vi "TX.vi"() -> ()   [LabVIEW 2020]
uses:
  AppData/Local/Programs/Python/Python35-32/Control 1.ctl
  <vilib>/Analysis/2dsp.llb/1D Convolution (DBL).vi
  <vilib>/Analysis/baseanly.llb/Quick Scale 1D.vi
  <vilib>/addons/Modulation/Analog/support/mod_Set Error Source.vi
  <vilib>/Enthought/Python Integration Toolkit/api/Unpack Int Array.vi
  <vilib>/addons/Modulation/Digital/Support/Common/Validators/mod_Generate Filter Coefficients Validate.vi
  <vilib>/addons/Modulation/Digital/General/subVIs/mod_Generate Filter Coefficients.vi
  <vilib>/Analysis/2dsp.llb/Upsample (DBL).vi
  <vilib>/measure/maspectr.llb/FFT Power Spectrum and PSD for 1 Chan (CDB).vi
  <instrlib>/niUSRP/niUSRP Write Tx Data (CDB Cluster).vi
  <vilib>/Analysis/NI_AALPro.lvlib
  <vilib>/measure/NI_MAPro.lvlib
  <vilib>/addons/Modulation/niDMT.lvlib
  <vilib>/Analysis/NI_AALBase.lvlib
  <vilib>/Enthought/Python Integration Toolkit/Python Integration Toolkit.lvlib
panel:
  in  "file path (use dialog)":path=path "C:/Users/ira_1/AppData/Local/Programs/Python/Python35-32/samples.txt"
  in  "Write sample file":bool
  in  "Timeout":dbl=10.0
  in  "Stop":bool
  in  "stop":bool
  in  "active antenna":string="TX1"
  out "Waveform Graph 2":cluster{"f0":dbl, "df":dbl, "magnitude":dbl[]}(graph)
  out "Waveform Graph":waveform(dbl)(graph)
  in  "averaging parameters":T1={"averaging mode"=enum."No averaging", "weighting mode"=enum."Exponential", "number of averages"=10} {"number of averages" min=1}
  in  "Delay":dbl
  out "error out":errorcluster
  out "Value":i32[](array[numeric])
  out "Кол-во символов":dbl
  in  "speed symbols(sym/sec)":dbl=1023000.0
  in  "NKA id":dbl=1.0
  in  "Doppler":dbl
  out "coerced gain(dB":dbl
  out "coerced carrier frequency":dbl
  out "coerced IQ rate":dbl
  in  "USRP name":T2="B200"
  in  "IQ rate(дискретизацтя)":dbl=4092000.0
  in  "Gain(dB)":dbl=-10.0
  in  "Freq":dbl=1575450000.0
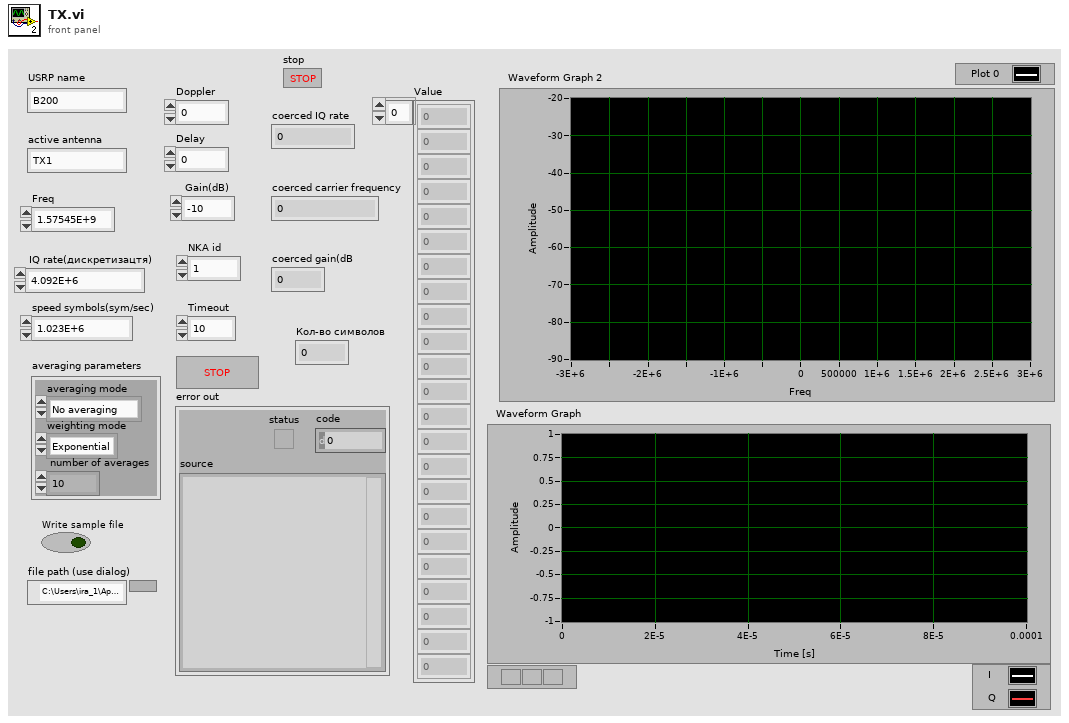
[diagram p1: front panel]
types:
  T1 = cluster{"averaging mode":enum16{"No averaging", "Vector averaging", "RMS averaging", "Peak hold"}, "weighting mode":enum16{"Linear", "Exponential"}, "number of averages":u32}
  T2 = typedef "Control 1.ctl" = string
  T3 = enum16{"none", "Raised Cosine", "Root Raised Cos", "Gaussian"}
  T4 = enum16{"FSK", "PSK", "QAM", "MSK", "PAM", "ASK", "CPM"}
  T5 = enum16{"open", "replace", "create", "open or create", "replace or create", "replace or create with confirmation"}
  T6 = typedef "Python Integration Toolkit.lvlib/Session ID.ctl" = u64
  T7 = typedef "Python Integration Toolkit.lvlib/Python Objects.ctl" = variant
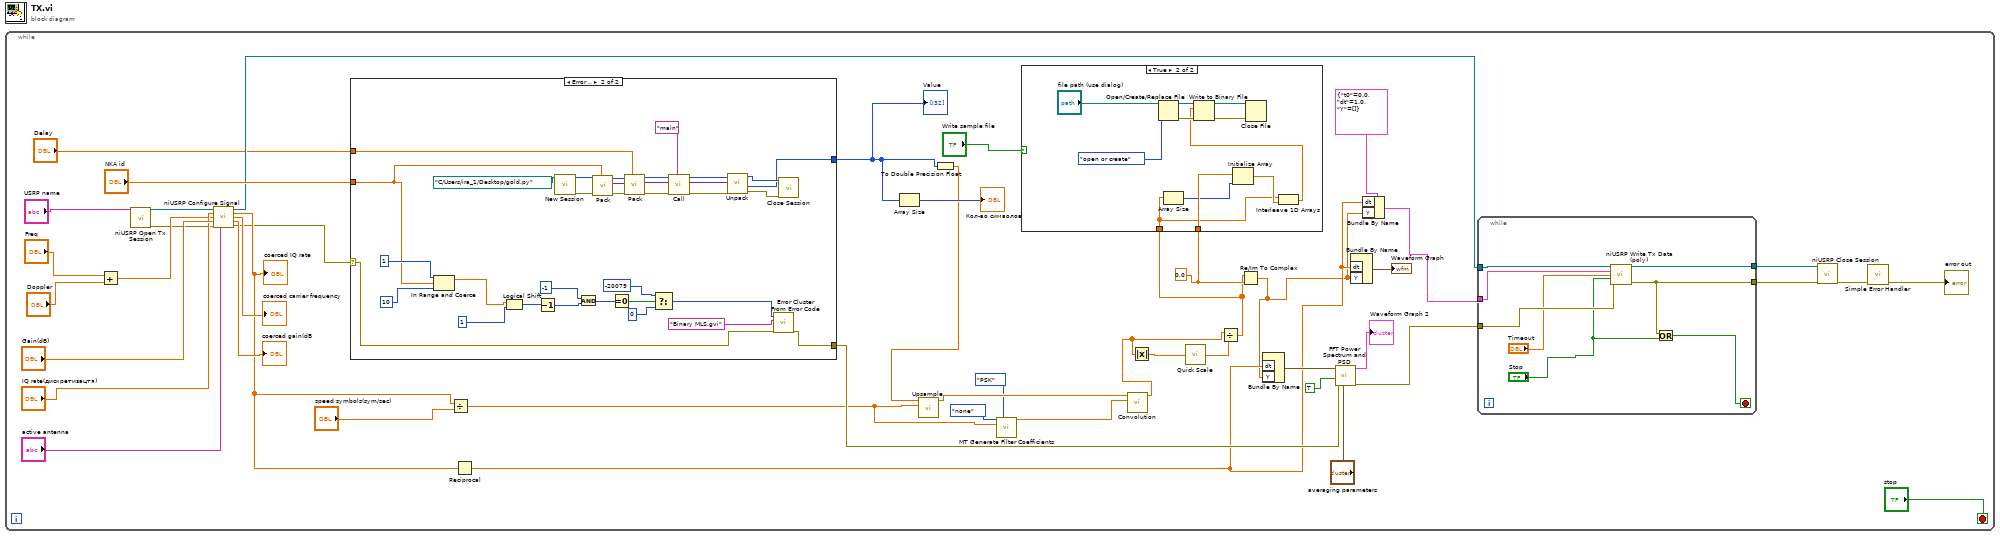
[diagram p0: block diagram]
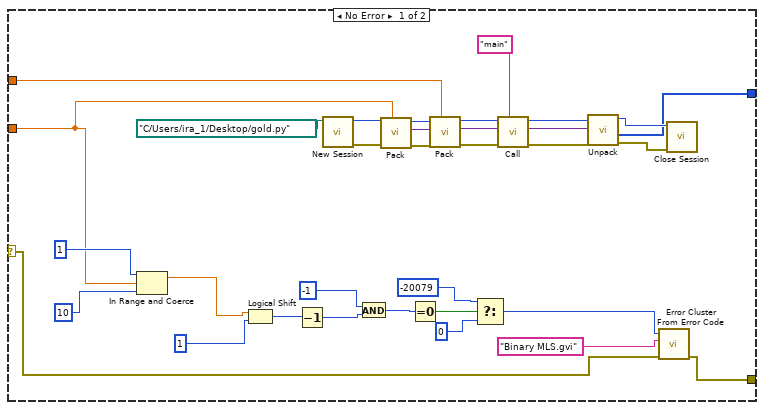
[diagram p3: hidden frame]
diagram:
  n1 = while {
    stop <- "stop" stop-if-true
    w3 = 0.0
    n2 = Add(x="Freq", y="Doppler") -> (x+y=w39:dbl)
    n3 = call <instrlib>:"niUSRP Open Tx Session.vi"("device names"="USRP name") -> ("session handle out"=w46:refnum<k15>, "error out"=w13:errorcluster)  [unwired: 13 in]
    n4 = call <instrlib>:"niUSRP Configure Signal.vi"("session handle"=w46, "IQ rate"="IQ rate(дискретизацтя)", "carrier frequency"=w39, "gain"="Gain(dB)", "error in (no error)"=w13, "active antenna"="active antenna") -> ("session handle out"=w25:refnum<k15>, "coerced IQ rate"=w36:dbl, "coerced carrier frequency"=→"coerced carrier frequency":dbl, "coerced gain"=→"coerced gain(dB":dbl, "error out"=w8:errorcluster)  [unwired: 5 in]
    "coerced IQ rate" <- w36
    n5 = case shown="Error .." w8 {
      selector: w8 -> [w67 w100]
      tunnel: "NKA id" -> [w69 w102]
      tunnel: [w86 w119] -> w32
      tunnel: [w75 w108] -> w34
      tunnel: "Delay" -> [w68 w101]
      frame No Error {
        n6 = In Range and Coerce(upper limit=1, x=w69, lower limit=10) -> (coerced(x)=w96:dbl)  [unwired: 1 out]
        n7 = Logical Shift(y=w96, x=1) -> (x << y=w95:i32)
        n8 = Decrement(x=w95) -> (x-1=w94:i32)
        n9 = call <vilib>:"New Session.vi"("Path to Python Module (.py File)"=path "C:/Users/ira_1/Desktop/gold.py") -> ("error out"=w73:errorcluster, "Session ID out"=w74:T6)  [unwired: 9 in]
        n10 = And(x=-1, y=w94) -> (x .and. y?=w92:i32)
        n11 = call <vilib>:"Pack.vi"("Argument"=w69, "error in (no error)"=w73, "Session ID"=w74) -> ("error out"=w72:errorcluster, "Python Object References Out"=w70:T7, "Session ID out"=w71:T6)  [unwired: 6 in]
        n12 = Equal To 0?(x=w92) -> (x = 0?=w91:bool)
        n13 = call <vilib>:"Pack.vi"("Argument"=w68, "error in (no error)"=w72, "Python Object References In"=w70, "Session ID"=w71) -> ("error out"=w79:errorcluster, "Python Object References Out"=w76:T7, "Session ID out"=w85:T6)  [unwired: 5 in]
        n14 = Select(t=-20079, s=w91, f=0) -> (s? t:f=w87:i32)
        n15 = call <vilib>:"Call.vi"("Function or Method Name"="main", "error in (no error)"=w79, "Python Object References In"=w76, "Session ID"=w85) -> ("error out"=w80:errorcluster, "Python Object References Out"=w81:T7, "Session ID out"=w84:T6)  [unwired: 5 in]
        n16 = call-poly <vilib>:"Unpack.vi"("error in (no error)"=w80, "Python Object References In"=w81, "Session ID"=w84) -> ("error out"=w82:errorcluster, "Value"=w75:i32[], "Session ID out"=w83:T6)  [unwired: 5 in, 1 out]
        n17 = call <vilib>:"Error Cluster From Error Code.vi"("error in (no error)"=w67, "error message (\"\")"="Binary MLS.gvi", "error code (0)"=w87) -> ("error out"=w86:errorcluster)  [unwired: 6 in]
        n18 = call <vilib>:"Close Session.vi"("error in (no error)"=w82, "Session ID"=w83) -> ()  [unwired: 9 in, 1 out]
      }
      frame Error {
        n19 = In Range and Coerce(upper limit=1, x=w102, lower limit=10) -> (coerced(x)=w129:dbl)  [unwired: 1 out]
        n20 = Logical Shift(y=w129, x=1) -> (x << y=w128:i32)
        n21 = Decrement(x=w128) -> (x-1=w127:i32)
        n22 = call <vilib>:"New Session.vi"("Path to Python Module (.py File)"=path "C:/Users/ira_1/Desktop/gold.py") -> ("error out"=w106:errorcluster, "Session ID out"=w107:T6)  [unwired: 9 in]
        n23 = And(x=-1, y=w127) -> (x .and. y?=w125:i32)
        n24 = call <vilib>:"Pack.vi"("Argument"=w102, "error in (no error)"=w106, "Session ID"=w107) -> ("error out"=w105:errorcluster, "Python Object References Out"=w103:T7, "Session ID out"=w104:T6)  [unwired: 6 in]
        n25 = Equal To 0?(x=w125) -> (x = 0?=w124:bool)
        n26 = call <vilib>:"Pack.vi"("Argument"=w101, "error in (no error)"=w105, "Python Object References In"=w103, "Session ID"=w104) -> ("error out"=w112:errorcluster, "Python Object References Out"=w109:T7, "Session ID out"=w118:T6)  [unwired: 5 in]
        n27 = Select(t=-20079, s=w124, f=0) -> (s? t:f=w120:i32)
        n28 = call <vilib>:"Call.vi"("Function or Method Name"="main", "error in (no error)"=w112, "Python Object References In"=w109, "Session ID"=w118) -> ("error out"=w113:errorcluster, "Python Object References Out"=w114:T7, "Session ID out"=w117:T6)  [unwired: 5 in]
        n29 = call-poly <vilib>:"Unpack.vi"("error in (no error)"=w113, "Python Object References In"=w114, "Session ID"=w117) -> ("error out"=w115:errorcluster, "Value"=w108:i32[], "Session ID out"=w116:T6)  [unwired: 5 in, 1 out]
        n30 = call <vilib>:"Error Cluster From Error Code.vi"("error in (no error)"=w100, "error message (\"\")"="Binary MLS.gvi", "error code (0)"=w120) -> ("error out"=w119:errorcluster)  [unwired: 6 in]
        n31 = call <vilib>:"Close Session.vi"("error in (no error)"=w115, "Session ID"=w116) -> ()  [unwired: 9 in, 1 out]
      }
    }
    "Value" <- w34
    n32 = Divide(x=w36, y="speed symbols(sym/sec)") -> (x/y=w23:dbl)
    n33 = Reciprocal(x=w36) -> (1/x=w12:dbl)
    n34 = Array Size(array=w34) -> (size(s)=→"Кол-во символов":i32)
    n35 = To Double Precision Float(number=w34) -> (double precision float=w33:dbl[])
    n36 = call-poly <vilib>:"Upsample.vi"("upsampling factor"=w23, "X"=w33) -> ("Upsampled Array"=w21:dbl[])  [unwired: 8 in, 1 out]
    n37 = call <vilib>:"MT Generate Filter Coefficients.vi"("pulse shaping filter (none)"=T3."none", "modulation type"=T4."PSK", "pulse shaping samples per symbol (16)"=w23) -> ("pulse shaping filter coefficients"=w22:dbl[])  [unwired: 10 in, 2 out]
    n38 = call-poly <vilib>:"Convolution.vi"("Y"=w22, "X"=w21) -> ("X * Y"=w18:dbl[])  [unwired: 8 in, 1 out]
    n39 = Absolute Value(x=w18) -> (abs(x)=w15:dbl[])
    n40 = call-poly <vilib>:"Quick Scale.vi"("X"=w15) -> ("max|X|"=w14:dbl)  [unwired: 2 out]
    n41 = Divide(x=w18, y=w14) -> (x/y=w2:dbl[])
    n42 = case shown="True" "Write sample file" {
      tunnel: w3 -> [_ w58]
      tunnel: w2 -> [_ w50]
      frame False {
      }
      frame True {
        n43 = Open/Create/Replace File(file path (use dialog)="file path (use dialog)", operation (0:open)=T5."open or create") -> (refnum out=w55:refnum<file>, error out=w54:errorcluster)  [unwired: 4 in, 1 out]
        n44 = Array Size(array=w50) -> (size(s)=w57:i32)
        n45 = Initialize Array(w58, w57) -> (w56:dbl[])
        n46 = Interleave 1D Arrays(w50, w56) -> (w53:dbl[])
        n47 = Write to Binary File(file (use dialog)=w55, data=w53, error in=w54) -> (refnum out=w51:refnum<file>, error out=w52:errorcluster)  [unwired: 3 in, 1 out]
        n48 = Close File(refnum=w51, error in=w52) -> ()  [unwired: 2 out]
      }
    }
    n49 = Re/Im To Complex(1:w3, 2:w2) -> (0:w4:cdb[])
    n50 = Bundle By Name("dt"=w12, "Y"=w4) -> (w17:waveform(cdb))  [unwired: 1 in]
    n51 = call-poly <vilib>:"FFT Power Spectrum and PSD.vi"("averaging parameters"="averaging parameters", "error in (no error)"=w32, "dB On (F)"=TRUE, "time signal"=w17) -> ("error out"=w30:errorcluster, "Power Spectrum / PSD"=→"Waveform Graph 2":cluster{"f0":dbl, "df":dbl, "magnitude":dbl[]})  [unwired: 4 in, 2 out]
    n52 = Bundle By Name("dt"=w12, "Y"=w4) -> (→"Waveform Graph":waveform(cdb))  [unwired: 1 in]
    n53 = Bundle By Name(cluster=cluster{"t0":dbl, "dt":dbl, "Y":cdb[]} {"t0"=0.0, "dt"=1.0, "Y"=[]} ("data"), "dt"=w12, "Y"=w4) -> (w11:cluster{"t0":dbl, "dt":dbl, "Y":cdb[]})
    n54 = while {
      tunnel: w25 -> [w62]
      tunnel: [w66] -> w29
      tunnel: [w64] -> w28
      tunnel: w30 -> [w65]
      tunnel: w11 -> [w61]
      stop <- w63 stop-if-true
      n55 = call-poly <instrlib>:"niUSRP Write Tx Data (poly).vi"("session handle"=w62, "data"=w61, "timeout"="Timeout", "end of data?"="Stop", "error in (no error)"=w65) -> ("session handle out"=w66:refnum<k15>, "error out"=w64:errorcluster)  [unwired: 9 in]
      n56 = Or(x=w64, y="Stop") -> (x .or. y?=w63:bool)
    }
    n57 = call <instrlib>:"niUSRP Close Session.vi"("session handle"=w29, "error in (no error)"=w28) -> ("error out"=w27:errorcluster)  [unwired: 13 in]
    n58 = call <vilib>:"Simple Error Handler.vi"("error in (no error)"=w27) -> ("error out"=→"error out":errorcluster)  [unwired: 4 in, 4 out]
  }
